vi "Pre Launch Init.vi"(11 "CS++GUIActor in":refnum<class "CS++GUIActor.lvclass">) -> (0 "error out":errorcluster, 3 "CS++GUIActor out":refnum<class "CS++GUIActor.lvclass">)   [LabVIEW 2014, in "CS++GUIActor.lvlib" / "CS++GUIActor.lvclass"]
doc: "(<B>Filename</B>: Actor Framework.lvlib:Actor.lvclass:Pre Launch Init.vi)\n\nDefines behavior that occurs after the Launch Actor method is invoked but before the actor's Actor Core method begins running.\n\nThe Pre Launch Init method is guaranteed to finish before the Launch Actor method returns to its caller and before the actor itself receives any messages. Any references that the Pre Launch Init method obtains are guaranteed to have the same lifetime as the actor itself. Any errors that the Pre Launch Init method returns will abort the launch.\n\nBy default, this method does nothing. A descendant class may override it to define behavior."
uses:
  CS++GUIActor.lvclass
  Classes/CS++ProcessVariables/ProcessVariable/PV.lvclass
  CS++GUIActor.lvclass/CS++GUIActor.ctl
  CS++BaseActor/CS++BaseActor.lvclass
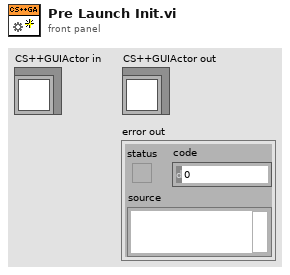
[diagram p1: front panel]
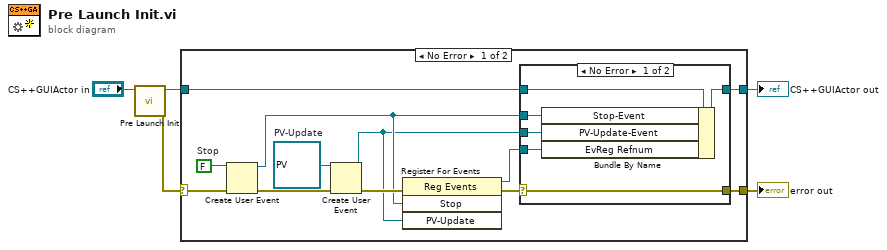
[diagram p0: block diagram]
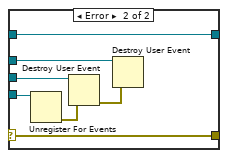
[diagram p2: hidden frame]
diagram:
  n1 = call-parent "Pre Launch Init.vi"("CS++BaseActor in"="CS++GUIActor in") -> ("error out"=w4:errorcluster, "CS++BaseActor out"=w3:refnum<class "CS++GUIActor.lvclass">)  [unwired: 9 in]
  n2 = case shown="No Error" w4 {
    selector: w4 -> [w15 w31]
    tunnel: w3 -> [w13 w32]
    tunnel: [w12 w32] -> w2
    tunnel: [w11 w31] -> w1
    frame No Error {
      w16 = refnum<class "PV.lvclass"> refnum  # PV-Update
      w17 = FALSE  # Stop
      n3 = Create User Event(user event datatype=w17, error in=w15) -> (user event=w8:refnum<user-event>, error out=w14:errorcluster)
      n4 = Create User Event(user event datatype=w16, error in=w14) -> (user event=w7:refnum<user-event>, error out=w10:errorcluster)
      n5 = register-events(error in=w10, w8, w7) -> (reference out=w6:refnum<event-registration>, error out=w9:errorcluster)  [unwired: 1 in]
      n6 = case shown="No Error" w9 {
        selector: w9 -> [w19 w27]
        tunnel: w8 -> [w23 w29]
        tunnel: w7 -> [w22 w30]
        tunnel: w13 -> [w21 w28]
        tunnel: [w20 w28] -> w12
        tunnel: [w19 w27] -> w11
        tunnel: w6 -> [w18 w26]
        frame No Error {
          n7 = Bundle By Name(cluster=w21, "Stop-Event"=w23, "PV-Update-Event"=w22, "EvReg Refnum"=w18) -> (w20:refnum<class "CS++GUIActor.lvclass">)
        }
        frame Error {
          n8 = Unregister For Events(event registration refnum=w26) -> (error out=w25:errorcluster)  [unwired: 1 in]
          n9 = Destroy User Event(user event=w30, error in=w25) -> (error out=w24:errorcluster)
          n10 = Destroy User Event(user event=w29, error in=w24) -> ()  [unwired: 1 out]
        }
      }
    }
    frame Error {
    }
  }
  "error out" <- w1
  "CS++GUIActor out" <- w2
